vi "Read Time.vi"(8 "error in (no error)":errorcluster, 11 "Test Case in":refnum<class "Test Case.lvclass">) -> (0 "error out":errorcluster, 2 "Time":dbl, 3 "Test Case out":refnum<class "Test Case.lvclass">)   [LabVIEW 2013, in "JUnit XML.lvlib" / "Test Case.lvclass"]
uses:
  Test Case.lvclass
  Test Case.lvclass/Test Case.ctl
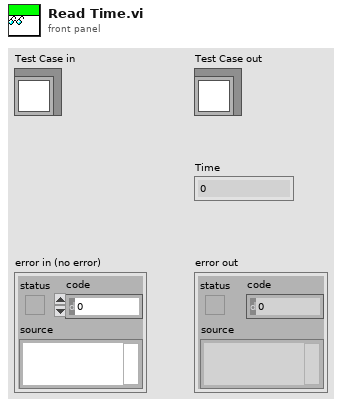
[diagram p1: front panel]
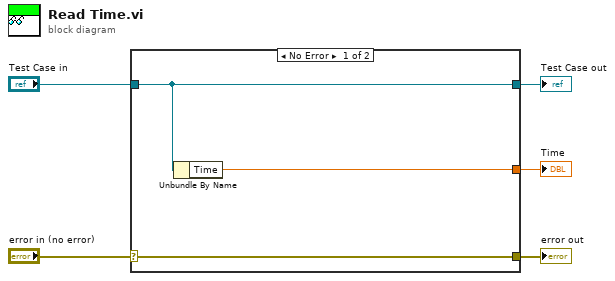
[diagram p0: block diagram]
diagram:
  n1 = case shown="No Error" "error in (no error)" {
    selector: "error in (no error)" -> [w8 w9]
    tunnel: [w8 w9] -> w4
    tunnel: [w7 w10] -> w2
    tunnel: "Test Case in" -> [w7 w10]
    tunnel: [w6 _] -> w1
    frame No Error {
      n2 = Unbundle By Name(w7) -> ("Time"=w6:dbl)
    }
    frame Error {
    }
  }
  "error out" <- w4
  "Test Case out" <- w2
  "Time" <- w1
